vi "Load Wavelength Data.vi"(10 "Calibration File":path=path "C:/Users/Michael/Documents/GitHub/CampenLab/data/calib_1.csv") -> (1 "Numeric":i32, 2 "Array":dbl[](array[numeric]), 3 "all rows":dbl[][](array[numeric]) format="%#_14g")   [LabVIEW 2019, in "Spectrometer Calibration.lvlib"]
uses:
  Spectrometer Calibration.lvlib
  <vilib>/Utility/file.llb/Read Delimited Spreadsheet (DBL).vi
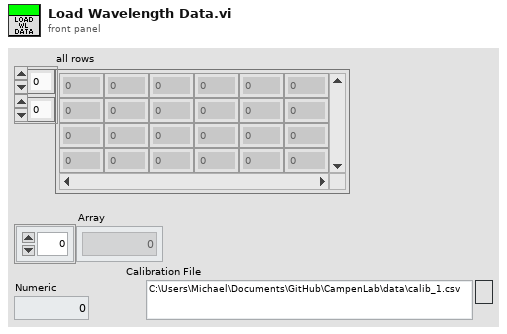
[diagram p1: front panel]
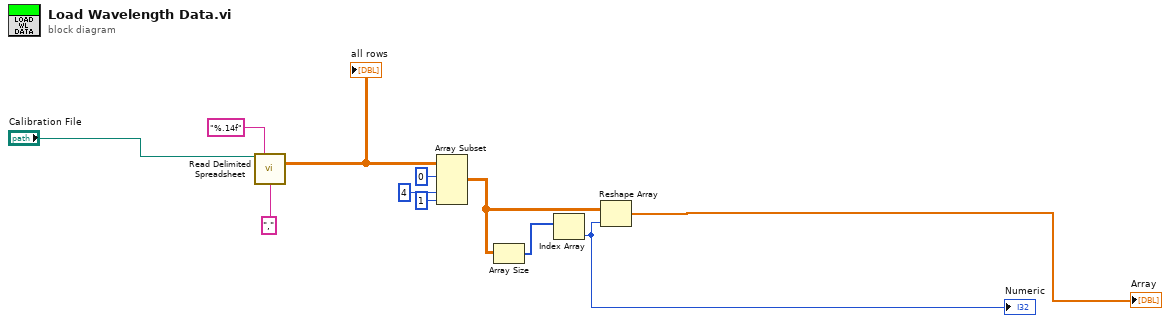
[diagram p0: block diagram]
diagram:
  n1 = call-poly <vilib>:"Read Delimited Spreadsheet.vi"("file path (dialog if empty)"="Calibration File", "format (%.3f)"="%.14f", "delimiter (\\t)"="," ("delimiter (\\t)")) -> ("all rows"=w4:dbl[][])  [unwired: 7 in, 5 out]
  "all rows" <- w4
  n2 = Array Subset(array=w4, index (row)=0 ("index"), index (col)=4 ("index"), length (col)=1 ("length")) -> (w8:dbl[][])  [unwired: 1 in]
  n3 = Array Size(array=w8) -> (size(s)=w7:i32[])
  n4 = Index Array(array=w7) -> (element=w10:i32)  [unwired: 1 in]
  "Numeric" <- w10
  n5 = Reshape Array(w8, w10) -> (→"Array":dbl[])
